vi "Exemple_Metrics_Average_Precision_Score.vi"() -> ()   [LabVIEW 2020]
uses:
  Objet/3 - Model selection and evaluation/3.3 - Metrics and scoring/average_precision_score/Average_Precision_Score.vi
panel:
  out "Score":string
  in  "average_precision_score":T1={"average"="macro", "pos_label"={"dtype_pos_label"="int", "pos_label"="1"}, "sample_weight"=[]}
  in  "y_score":string[][](array[string])=[["0,1"], ["0,4"], ["0,35"], ["0,8"]]
  in  "y_true":string[][](array[string])=[["0"], ["0"], ["1"], ["1"]]
  in  "error in":errorcluster caption="entrée d'erreur"
  out "error out":errorcluster caption="sortie d'erreur"
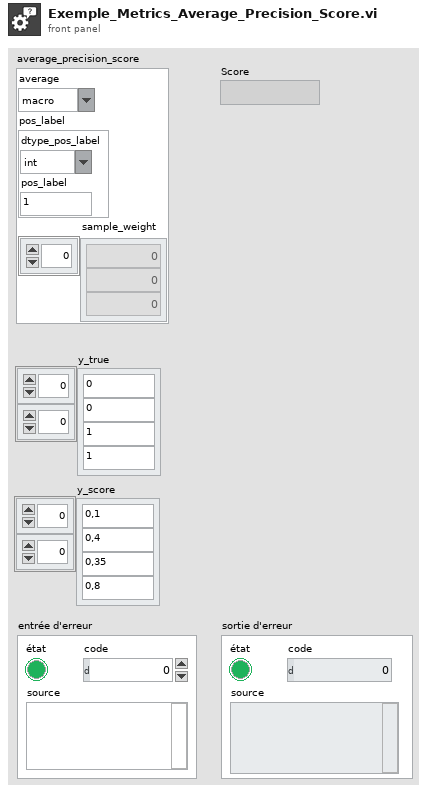
[diagram p1: front panel]
types:
  T1 = cluster{"average":string, "pos_label":cluster{"dtype_pos_label":string, "pos_label":string}, "sample_weight":dbl[]}
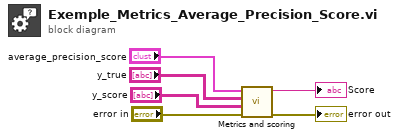
[diagram p0: block diagram]
diagram:
  n1 = call-poly "Metrics and scoring.vi"("error in (no error)"="error in", "y_score"="y_score", "y_true"="y_true", "average_precision_score"="average_precision_score") -> ("error out"=→"error out":errorcluster, "String Data"=→"Score":string)  [unwired: 6 in]
